vi "NT_LL_Read Raw.vi"(8 "error in (no error)":errorcluster, 10 "default value":string, 11 "subscribeHandle":u32) -> (0 "error out":errorcluster, 2 "time":i64, 3 "string":string)   [LabVIEW 2025]
uses:
  FRC_NetworkTablesLV.dll
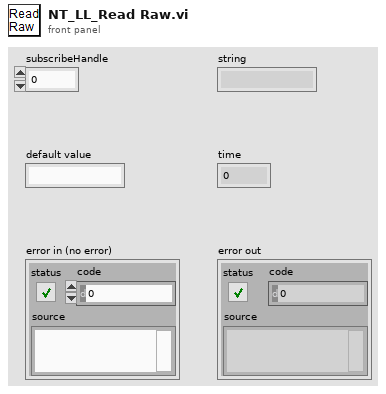
[diagram p1: front panel]
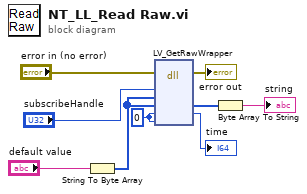
[diagram p0: block diagram]
diagram:
  w7 = i64 0 ("serverTime")
  n1 = String To Byte Array(string="default value") -> (unsigned byte array=w8:u8[])
  n2 = dll-call lib="FRC_NetworkTablesLV.*" fn="LV_GetRawWrapper"(error in="error in (no error)", "subscribeHandle"="subscribeHandle", "default"=w8, "value"=w8, "time"=w7, "serverTime"=w7) -> (error out=→"error out":errorcluster, "value"=w4:u8[], "time"=→"time":i64)  [unwired: 6 in, 1 out]
  n3 = Byte Array To String(unsigned byte array=w4) -> (string=→"string":string)
